vi "计算三角形重心.vi"(8 "Error In":errorcluster caption="错误输入", 11 "三角形":T1) -> (0 "Error Out":errorcluster caption="错误输出", 3 "重心":T2)   [LabVIEW 2012, in "几何工具.lvlib"]
uses:
  <vilib>/Utility/miscctls.llb/LVPointDoubleTypeDef.ctl
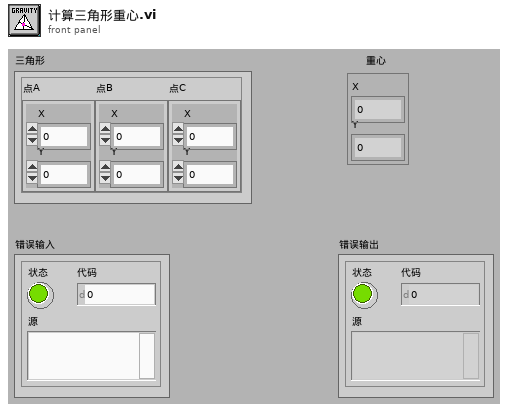
[diagram p1: front panel]
types:
  T1 = typedef "几何工具.lvlib/三角形.ctl" = cluster{"点A":T2, "点B":T2, "点C":T2}
  T2 = typedef "LVPointDoubleTypeDef.ctl" = cluster{"X":dbl, "Y":dbl}
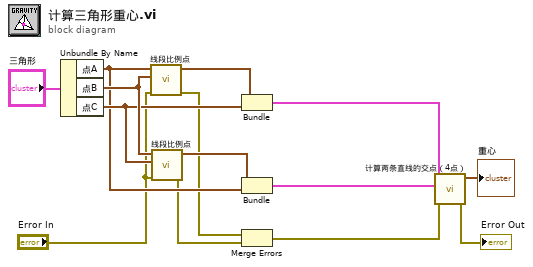
[diagram p0: block diagram]
diagram:
  n1 = Unbundle By Name("三角形") -> ("点A"=w8:T2, "点B"=w11:T2, "点C"=w10:T2)
  n2 = call "线段比例点.vi"("Error In"="Error In", "点B"=w11, "点A"=w8) -> ("Error Out"=w5:errorcluster, "比例点"=w13:T2)  [unwired: 7 in]
  n3 = call "线段比例点.vi"("Error In"="Error In", "点B"=w10, "点A"=w11) -> ("Error Out"=w3:errorcluster, "比例点"=w9:T2)  [unwired: 7 in]
  n4 = Bundle("比例点"=w13, "点C"=w10) -> (w12:cluster{"比例点":T2, "点C":T2})  [unwired: 1 in]
  n5 = Bundle("比例点"=w9, "点A"=w8) -> (w7:cluster{"比例点":T2, "点A":T2})  [unwired: 1 in]
  n6 = Merge Errors(w5, w3) -> (w2:errorcluster)
  n7 = call "计算两条直线的交点（4点）.vi"("Error In"=w2, "直线B"=w7, "直线A"=w12) -> ("Error Out"=→"Error Out":errorcluster, "交点"=→"重心":T2)  [unwired: 7 in]
